vi "空载判定.vi"(0 "曲线引用":refnum<vi>, 1 "空载判定条件":T1, 3 "错误输入":errorcluster) -> (7 "曲线引用输出":refnum<vi>, 8 "OK":bool, 10 "错误输出":errorcluster)   [LabVIEW 2018]
uses:
  <userlib>/_MGI/1D Array/MGI Average/MGI Average (DBL[]).vi
  Global_Variable/Global.vi
  Global_Variable/A180648.vi
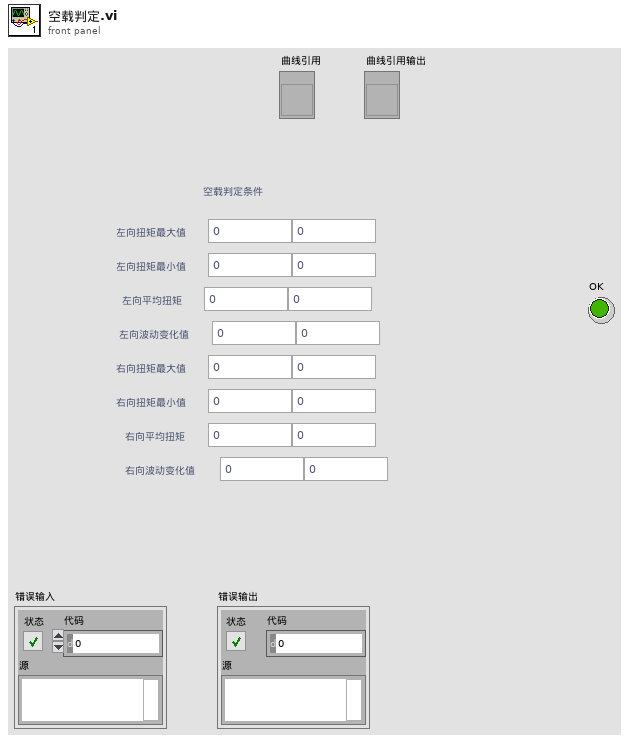
[diagram p1: front panel]
types:
  T1 = cluster{"左向扭矩最大值":cluster{"下限":dbl, "上限":dbl}, "左向扭矩最小值":cluster{"下限":dbl, "上限":dbl}, "  左向平均扭矩":cluster{"下限":dbl, "上限":dbl}, " 左向波动变化值":cluster{"下限":dbl, "上限":dbl}, "右向扭矩最大值":cluster{"下限":dbl, "上限":dbl}, "右向扭矩最小值":cluster{"下限":dbl, "上限":dbl}, "   右向平均扭矩":cluster{"下限":dbl, "上限":dbl}, "   右向波动变化值":cluster{"下限":dbl, "上限":dbl}}
  T2 = enum32{"空载", "功能", "力特性", "传感器特性", "电流特性", "振动NVH", "逆向空载", "完成"}
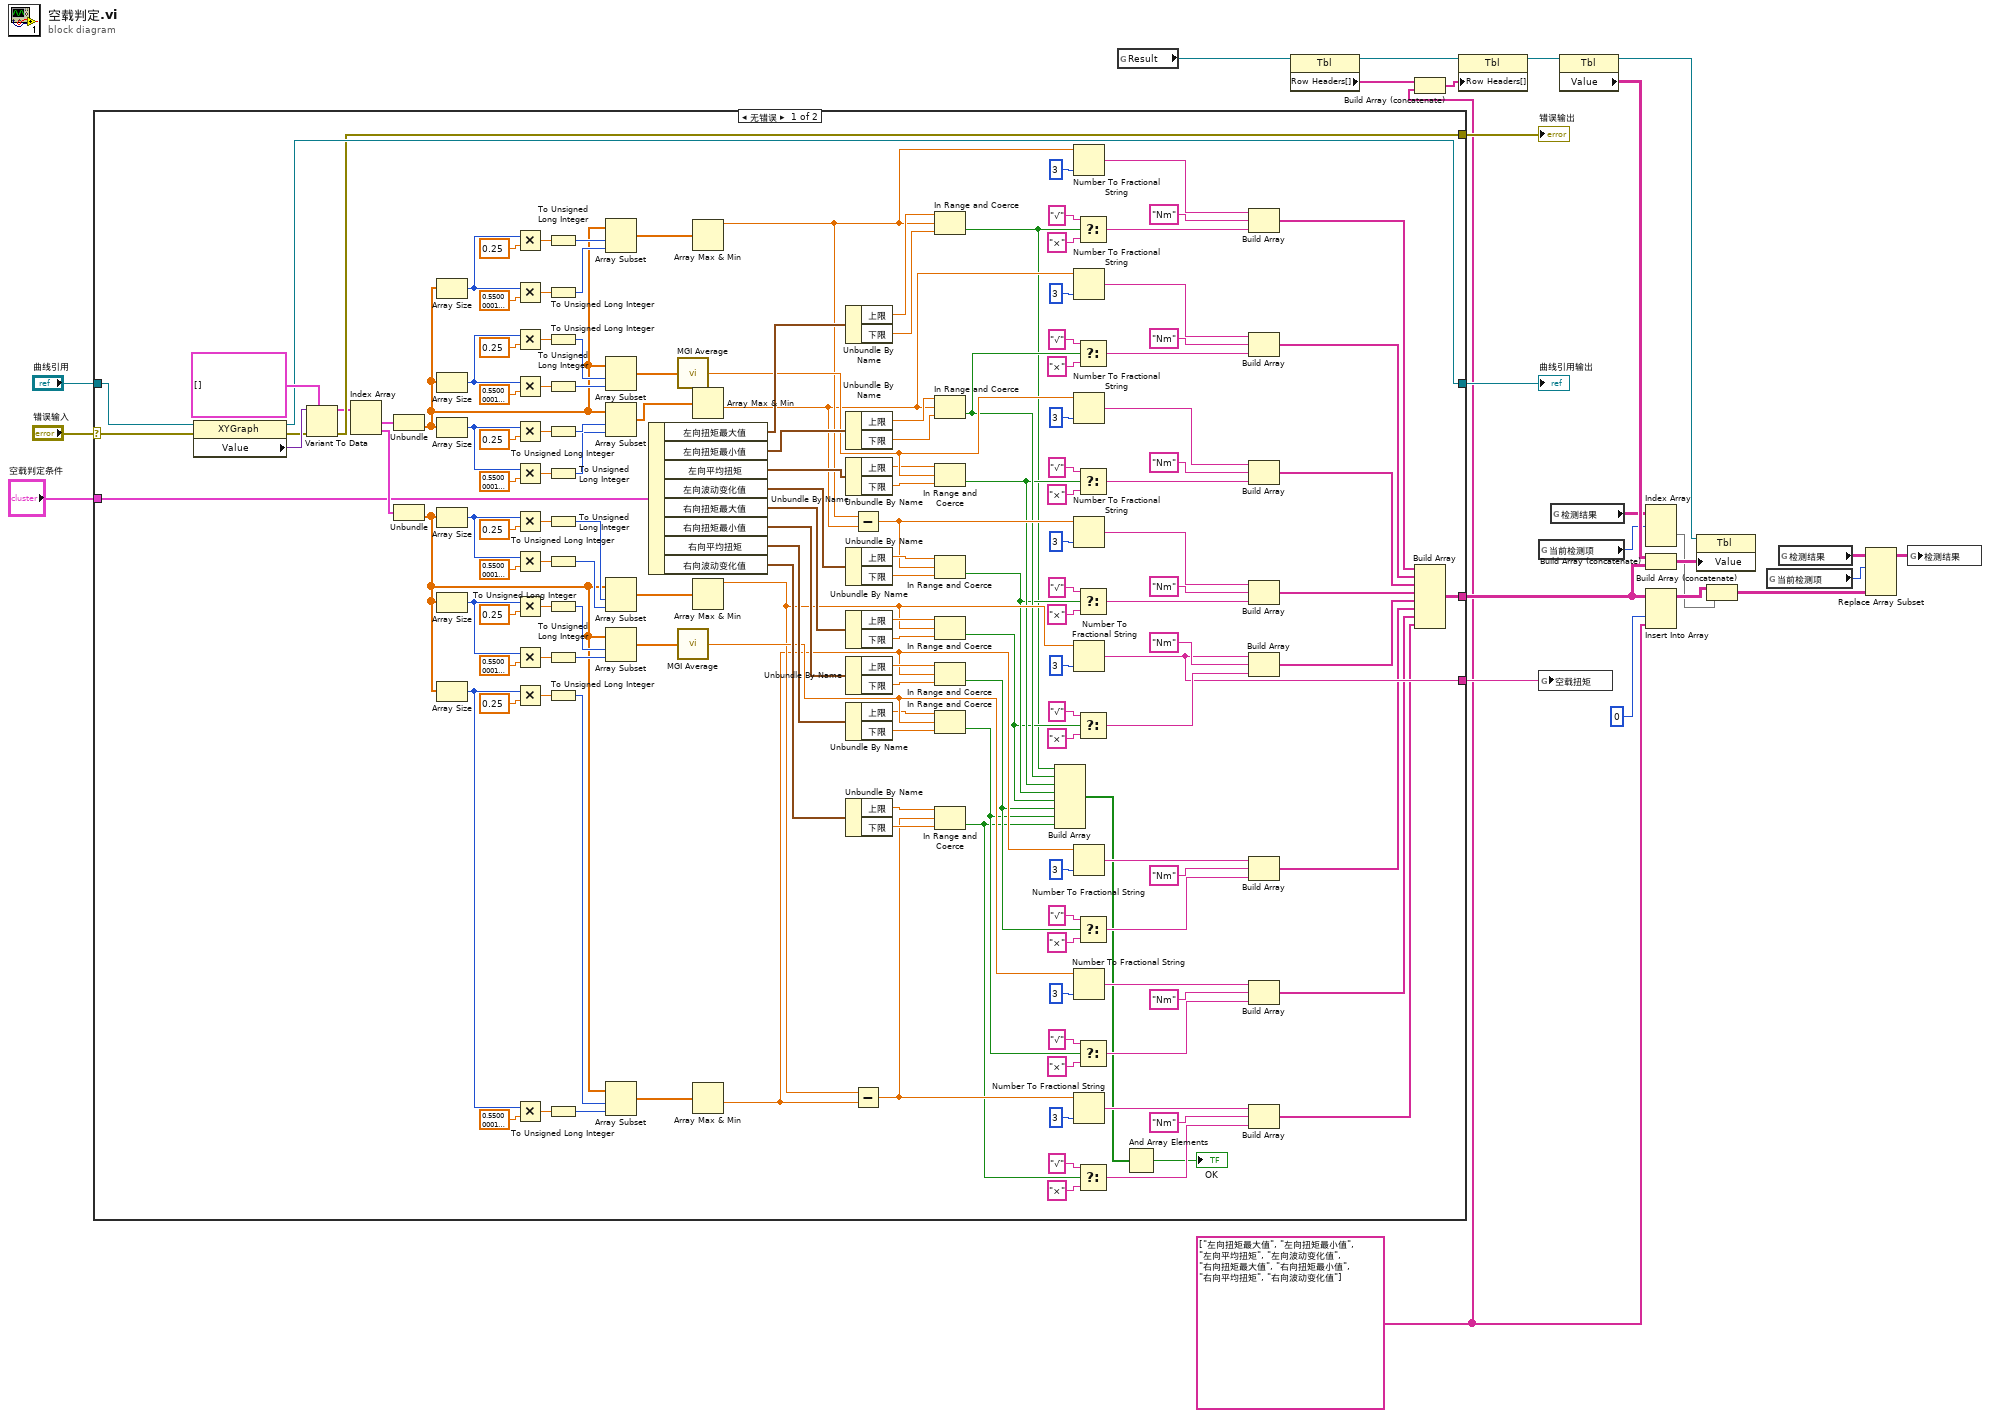
[diagram p0: block diagram]
diagram:
  w10 = string[] ["左向扭矩最大值", "左向扭矩最小值", "左向平均扭矩", "左向波动变化值", "右向扭矩最大值", "右向扭矩最小值", "右向平均扭矩", "右向波动变化值"] ("元素")
  n1 = case shown="无错误" "错误输入" {
    selector: "错误输入" -> [w183 w186]
    tunnel: [w179 w186] -> w24
    tunnel: "曲线引用" -> [w182 w187]
    tunnel: [w181 w187] -> w22
    tunnel: "空载判定条件" -> [w161 _]
    tunnel: [w129 _] -> w11
    tunnel: [w98 _] -> w12
    frame No Error {
      n2 = property class="XYGraph"(reference=w182, error in=w183) -> (reference out=w181:refnum<vi>, error out=w180:errorcluster, "Value"=w185:variant)
      n3 = Variant To Data(error in=w180, type=cluster{dbl[], dbl[]}[] [], Variant=w185) -> (data=w171:cluster{dbl[], dbl[]}[], error out=w179:errorcluster)
      n4 = Index Array(array=w171) -> (element #1=w170:cluster{dbl[], dbl[]}, element #2=w162:cluster{dbl[], dbl[]})  [unwired: 2 in]
      n5 = Unbundle(w170) -> (w71:dbl[])  [unwired: 1 out]
      n6 = Unbundle(w162) -> (w51:dbl[])  [unwired: 1 out]
      n7 = Array Size(array=w71) -> (size(s)=w121:i32)
      n8 = Array Size(array=w71) -> (size(s)=w172:i32)
      n9 = Array Size(array=w71) -> (size(s)=w122:i32)
      n10 = Array Size(array=w51) -> (size(s)=w100:i32)
      n11 = Array Size(array=w51) -> (size(s)=w169:i32)
      n12 = Array Size(array=w51) -> (size(s)=w99:i32)
      n13 = Multiply(x=w121, y=sgl 0.25) -> (x*y=w117:sgl)
      n14 = Multiply(x=w121, y=sgl 0.55) -> (x*y=w116:sgl)
      n15 = Multiply(x=w172, y=sgl 0.25) -> (x*y=w176:sgl)
      n16 = Multiply(x=w172, y=sgl 0.55) -> (x*y=w177:sgl)
      n17 = Multiply(x=w122, y=sgl 0.25) -> (x*y=w126:sgl)
      n18 = Multiply(x=w122, y=sgl 0.55) -> (x*y=w127:sgl)
      n19 = Multiply(x=w100, y=sgl 0.25) -> (x*y=w104:sgl)
      n20 = Multiply(x=w100, y=sgl 0.55) -> (x*y=w105:sgl)
      n21 = Multiply(x=w169, y=sgl 0.25) -> (x*y=w165:sgl)
      n22 = Multiply(x=w169, y=sgl 0.55) -> (x*y=w164:sgl)
      n23 = Multiply(x=w99, y=sgl 0.25) -> (x*y=w110:sgl)
      n24 = Multiply(x=w99, y=sgl 0.55) -> (x*y=w109:sgl)
      n25 = To Unsigned Long Integer(number=w117) -> (unsigned 32bit integer=w115:u32)
      n26 = To Unsigned Long Integer(number=w116) -> (unsigned 32bit integer=w120:u32)
      n27 = To Unsigned Long Integer(number=w176) -> (unsigned 32bit integer=w178:u32)
      n28 = To Unsigned Long Integer(number=w177) -> (unsigned 32bit integer=w173:u32)
      n29 = To Unsigned Long Integer(number=w126) -> (unsigned 32bit integer=w128:u32)
      n30 = To Unsigned Long Integer(number=w127) -> (unsigned 32bit integer=w123:u32)
      n31 = To Unsigned Long Integer(number=w104) -> (unsigned 32bit integer=w106:u32)
      n32 = To Unsigned Long Integer(number=w105) -> (unsigned 32bit integer=w101:u32)
      n33 = To Unsigned Long Integer(number=w165) -> (unsigned 32bit integer=w163:u32)
      n34 = To Unsigned Long Integer(number=w164) -> (unsigned 32bit integer=w168:u32)
      n35 = To Unsigned Long Integer(number=w110) -> (unsigned 32bit integer=w108:u32)
      n36 = To Unsigned Long Integer(number=w109) -> (unsigned 32bit integer=w113:u32)
      n37 = Array Subset(array=w71, index=w115, length=w120) -> (w70:dbl[])
      n38 = Array Subset(array=w71, index=w178, length=w173) -> (w27:dbl[])
      n39 = Array Subset(array=w71, index=w128, length=w123) -> (w114:dbl[])
      n40 = Array Subset(array=w51, index=w106, length=w101) -> (w50:dbl[])
      n41 = Array Subset(array=w51, index=w163, length=w168) -> (w26:dbl[])
      n42 = Array Subset(array=w51, index=w108, length=w113) -> (w107:dbl[])
      n43 = Unbundle By Name(w161) -> ("左向扭矩最大值"=w95:cluster{"下限":dbl, "上限":dbl}, "左向扭矩最小值"=w92:cluster{"下限":dbl, "上限":dbl}, "左向平均扭矩"=w97:cluster{"下限":dbl, "上限":dbl}, "左向波动变化值"=w93:cluster{"下限":dbl, "上限":dbl}, "右向扭矩最大值"=w94:cluster{"下限":dbl, "上限":dbl}, "右向扭矩最小值"=w91:cluster{"下限":dbl, "上限":dbl}, "右向平均扭矩"=w96:cluster{"下限":dbl, "上限":dbl}, "右向波动变化值"=w90:cluster{"下限":dbl, "上限":dbl})
      n44 = call-poly <userlib>:"MGI Average.vi"("Double[]"=w27) -> ("Average"=w63:dbl)  [unwired: 1 in]
      n45 = call-poly <userlib>:"MGI Average.vi"("Double[]"=w26) -> ("Average"=w47:dbl)  [unwired: 1 in]
      n46 = Array Max & Min(array=w70) -> (max value=w59:dbl)  [unwired: 3 out]
      n47 = Array Max & Min(array=w114) -> (min value=w58:dbl)  [unwired: 3 out]
      n48 = Array Max & Min(array=w50) -> (max value=w41:dbl)  [unwired: 3 out]
      n49 = Array Max & Min(array=w107) -> (min value=w40:dbl)  [unwired: 3 out]
      n50 = Unbundle By Name(w95) -> ("上限"=w69:dbl, "下限"=w68:dbl)
      n51 = Unbundle By Name(w92) -> ("上限"=w66:dbl, "下限"=w65:dbl)
      n52 = Unbundle By Name(w97) -> ("上限"=w62:dbl, "下限"=w61:dbl)
      n53 = Unbundle By Name(w93) -> ("上限"=w56:dbl, "下限"=w55:dbl)
      n54 = Unbundle By Name(w94) -> ("上限"=w53:dbl, "下限"=w52:dbl)
      n55 = Unbundle By Name(w91) -> ("上限"=w49:dbl, "下限"=w48:dbl)
      n56 = Unbundle By Name(w96) -> ("上限"=w46:dbl, "下限"=w45:dbl)
      n57 = Unbundle By Name(w90) -> ("上限"=w39:dbl, "下限"=w38:dbl)
      n58 = Subtract(x=w59, y=w58) -> (x-y=w54:dbl)
      n59 = Subtract(x=w41, y=w40) -> (x-y=w37:dbl)
      n60 = In Range and Coerce(upper limit=w69, x=w59, lower limit=w68) -> (In Range?=w30:bool)  [unwired: 1 out]
      n61 = In Range and Coerce(upper limit=w66, x=w58, lower limit=w65) -> (In Range?=w35:bool)  [unwired: 1 out]
      n62 = In Range and Coerce(upper limit=w62, x=w63, lower limit=w61) -> (In Range?=w34:bool)  [unwired: 1 out]
      n63 = In Range and Coerce(upper limit=w56, x=w54, lower limit=w55) -> (In Range?=w33:bool)  [unwired: 1 out]
      n64 = In Range and Coerce(upper limit=w53, x=w41, lower limit=w52) -> (In Range?=w32:bool)  [unwired: 1 out]
      n65 = In Range and Coerce(upper limit=w49, x=w40, lower limit=w48) -> (In Range?=w31:bool)  [unwired: 1 out]
      n66 = In Range and Coerce(upper limit=w46, x=w47, lower limit=w45) -> (In Range?=w29:bool)  [unwired: 1 out]
      n67 = In Range and Coerce(upper limit=w39, x=w37, lower limit=w38) -> (In Range?=w28:bool)  [unwired: 1 out]
      n68 = Build Array(w30, w35, w34, w33, w32, w31, w29, w28) -> (w131:bool[])
      n69 = Number To Fractional String(number=w59, precision (6)=i16 3 ("精度(6)")) -> (F-format string=w73:string)  [unwired: 2 in]
      n70 = Number To Fractional String(number=w58, precision (6)=i16 3 ("精度(6)")) -> (F-format string=w82:string)  [unwired: 2 in]
      n71 = Number To Fractional String(number=w63, precision (6)=i16 3 ("精度(6)")) -> (F-format string=w85:string)  [unwired: 2 in]
      n72 = Number To Fractional String(number=w54, precision (6)=i16 3 ("精度(6)")) -> (F-format string=w159:string)  [unwired: 2 in]
      n73 = Number To Fractional String(number=w41, precision (6)=i16 3 ("精度(6)")) -> (F-format string=w98:string)  [unwired: 2 in]
      n74 = Number To Fractional String(number=w40, precision (6)=i16 3 ("精度(6)")) -> (F-format string=w136:string)  [unwired: 2 in]
      n75 = Number To Fractional String(number=w47, precision (6)=i16 3 ("精度(6)")) -> (F-format string=w150:string)  [unwired: 2 in]
      n76 = Number To Fractional String(number=w37, precision (6)=i16 3 ("精度(6)")) -> (F-format string=w139:string)  [unwired: 2 in]
      n77 = Select(t="√", s=w30, f="×") -> (s? t:f=w77:string)
      n78 = Select(t="√", s=w35, f="×") -> (s? t:f=w78:string)
      n79 = Select(t="√", s=w34, f="×") -> (s? t:f=w89:string)
      n80 = Select(t="√", s=w33, f="×") -> (s? t:f=w155:string)
      n81 = Select(t="√", s=w32, f="×") -> (s? t:f=w144:string)
      n82 = Select(t="√", s=w31, f="×") -> (s? t:f=w132:string)
      n83 = Select(t="√", s=w29, f="×") -> (s? t:f=w154:string)
      n84 = Select(t="√", s=w28, f="×") -> (s? t:f=w143:string)
      n85 = And Array Elements(Boolean array=w131) -> (logical AND=→"OK":bool)
      n86 = Build Array(w73, "Nm" ("元素"), w77) -> (w67:string[])
      n87 = Build Array(w82, "Nm" ("元素"), w78) -> (w64:string[])
      n88 = Build Array(w85, "Nm" ("元素"), w89) -> (w60:string[])
      n89 = Build Array(w159, "Nm" ("元素"), w155) -> (w57:string[])
      n90 = Build Array(w98, "Nm" ("元素"), w144) -> (w44:string[])
      n91 = Build Array(w136, "Nm" ("元素"), w132) -> (w43:string[])
      n92 = Build Array(w150, "Nm" ("元素"), w154) -> (w42:string[])
      n93 = Build Array(w139, "Nm" ("元素"), w143) -> (w36:string[])
      n94 = Build Array(w67, w64, w60, w57, w44, w43, w42, w36) -> (w129:string[][])
    }
    frame Error {
    }
  }
  "错误输出" <- w24
  "曲线引用输出" <- w22
  n95 = global read "Global.vi" "Result"() -> (w20:refnum<vi>)
  n96 = property class="Tbl"(reference=w20) -> (reference out=w17:refnum<vi>, "Row Headers[]"=w19:string[])  [unwired: 1 in, 1 out]
  n97 = Build Array (concatenate)(w19, w10) -> (w18:string[])
  n98 = property class="Tbl"(reference=w17, "Row Headers[]"=w18) -> (reference out=w16:refnum<vi>)  [unwired: 1 in, 1 out]
  n99 = global read "A180648.vi" "当前检测项"() -> (w4:T2)
  n100 = global write "检测结果.vi" "空载扭矩"(w12) -> ()
  n101 = global read "A180648.vi" "检测结果"() -> (w5:string[][][])
  n102 = property class="Tbl"(reference=w16) -> (reference out=w15:refnum<vi>, "Value"=w14:string[][])  [unwired: 1 in, 1 out]
  n103 = Index Array(array=w5, index (dim 0)=w4) -> (element=w1:string[][])  [unwired: 2 in]
  n104 = Build Array (concatenate)(w14, w11) -> (w13:string[][])
  n105 = Insert Into Array(array=w11, index (col)=0 ("禁用的索引 (列)"), new element=w10) -> (w2:string[][])  [unwired: 1 in]
  n106 = property class="Tbl"(reference=w15, "Value"=w13) -> ()  [unwired: 1 in, 2 out]
  n107 = Build Array (concatenate)(w2, w1) -> (w3:string[][])
  n108 = global read "A180648.vi" "当前检测项"() -> (w7:T2)
  n109 = global read "A180648.vi" "检测结果"() -> (w8:string[][][])
  n110 = Replace Array Subset(array=w8, new element=w3, index (dim 0)=w7) -> (w6:string[][][])  [unwired: 2 in]
  n111 = global write "A180648.vi" "检测结果"(w6) -> ()
